vi "NI ELVIS - Initialize Wrap.vi"(8 "error in":errorcluster, 11 "Device Name":tag) -> (0 "error out":errorcluster, 2 "Device Name (out)":tag, 3 "NI ELVIS Refnum":T1)   [LabVIEW 2010]
uses:
  <instrlib>/NI ELVIS Traditional/NI ELVIS - RSCMAN.llb/ELVIS RSCMAN - NI ELVIS Refnum.ctl
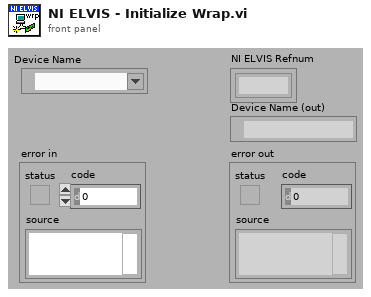
[diagram p1: front panel]
types:
  T1 = typedef "ELVIS RSCMAN - NI ELVIS Refnum.ctl" = refnum<k1>
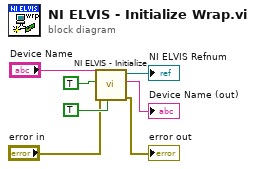
[diagram p0: block diagram]
diagram:
  n1 = call <instrlib>:"NI ELVIS - Initialize.vi"("show popup?"=TRUE, "error in"="error in", "Global Reset"=TRUE, "Device Name"="Device Name") -> ("error out"=→"error out":errorcluster, "Device Name (out)"=→"Device Name (out)":tag, "NI ELVIS Refnum"=→"NI ELVIS Refnum":T1)  [unwired: 4 in, 1 out]
